vi "Send To Created.vi"(4 "Is Priority":bool, 6 "Alias":string, 7 "Actor in":refnum<class "Actor.lvclass">) -> (0 "Error out":errorcluster)   [LabVIEW 2025, in "_Template.lvlib" / "Templates.lvlib" / "TEMPLATE Msg.lvlib"]
uses:
  TEMPLATE Msg.lvlib
  jettl/jettl/Actor/Actor/Actor.lvclass
  TEMPLATE Msg/TEMPLATE Msg.lvclass
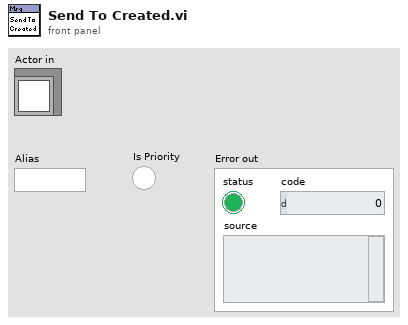
[diagram p1: front panel]
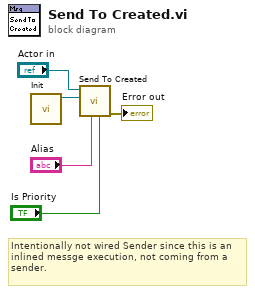
[diagram p0: block diagram]
diagram:
  # "Intentionally not wired Sender since this is an inlined messge execution, not coming from a sender."
  n1 = call "Init.vi"() -> ("TEMPLATE Msg out"=w1:refnum<class "TEMPLATE Msg.lvclass">)  [unwired: 11 in]
  n2 = call-dynamic "Send To Created.vi"("Is Priority"="Is Priority", "Alias"="Alias", "Msg"=w1, "Actor in"="Actor in") -> ("Error out"=→"Error out":errorcluster)  [unwired: 7 in]
